vi "cSM.vi"(8 "Error in":errorcluster) -> (0 "Error out":errorcluster)   [LabVIEW 2021, in "EDT VIE.lvlib"]
uses:
  EDT VIE.lvlib
panel:
  out "Current State":string
  out "Previous State":string
  in  "Tab Control":enum32{"Main", "Misc"}(tab)
  out "itr":i32
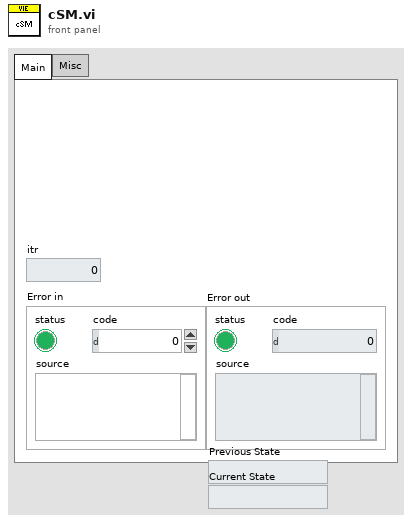
[diagram p1: front panel]
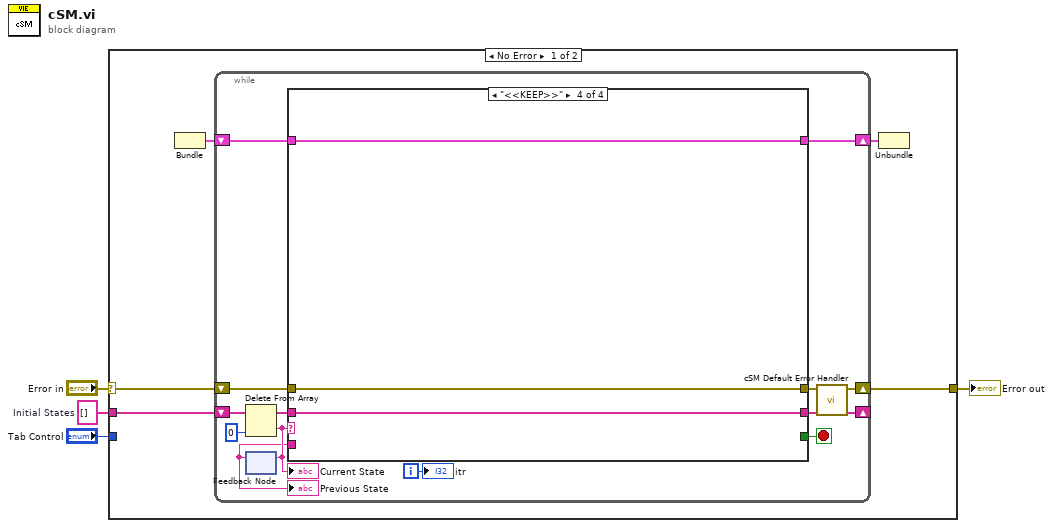
[diagram p0: block diagram]
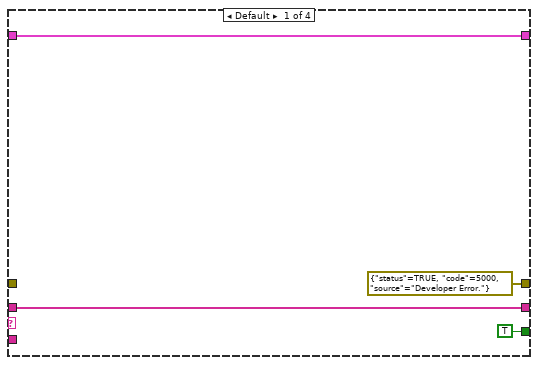
[diagram p2: hidden frame]
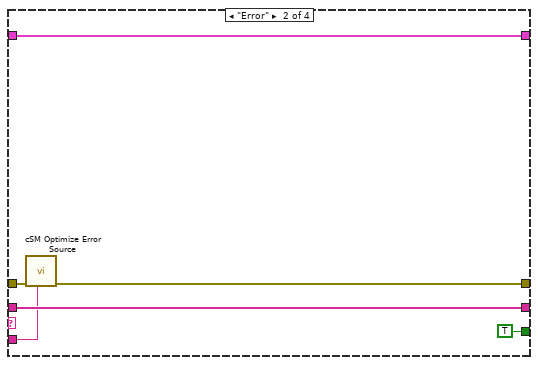
[diagram p3: hidden frame]
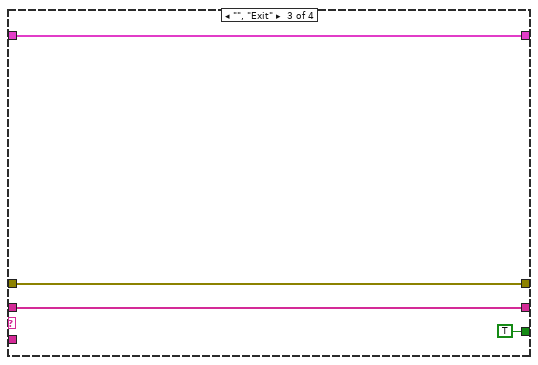
[diagram p4: hidden frame]
diagram:
  w4 = string[] []  # Initial States
  n1 = case shown="No Error" "Error in" {
    selector: "Error in" -> [w7 w41]
    tunnel: w4 -> [w9 _]
    tunnel: [w8 w41] -> w2
    tunnel: "Tab Control" -> [_ _]
    frame No Error {
      n2 = Bundle() -> (w6:cluster{void, void})  [unwired: 3 in]
      n3 = while {
        shift-right: [w10] -> _
        shift-left: w9 -> [w23]
        shift-right: [w12] -> w8
        shift-left: w7 -> [w20]
        shift-right: [w14] -> w5
        shift-left: w6 -> [w15]
        i -> [w21]
        stop <- w19 stop-if-true
        n4 = Delete From Array(array=w23, index=0) -> (deleted portion=w17:string, array with subset deleted=w22:string[])  [unwired: 1 in]
        "Current State" <- w17
        n5 = feedback #1() -> (w16:string)  [unwired: 1 in]
        "Previous State" <- w16
        n6 = feedback-in #1(w17) -> ()
        n7 = case shown="\"<<KEEP>>\"" w17 {
          tunnel: [w25 w33 w37 w40] -> w11
          tunnel: w22 -> [w25 w33 w37 w40]
          tunnel: w20 -> [_ w31 w36 w39]
          tunnel: [errorcluster {"status"=TRUE, "code"=5000, "source"="Developer Error."} ("error in") w30 w36 w39] -> w13
          tunnel: [TRUE TRUE TRUE _] -> w19
          tunnel: w16 -> [_ w29 _ _]
          tunnel: w15 -> [w24 w28 w34 w38]
          tunnel: [w24 w28 w34 w38] -> w14
          frame Default {
          }
          frame "Error" {
            n8 = call "cSM Optimize Error Source.vi"("Previous State"=w29, "Error in"=w31) -> ("Error out"=w30:errorcluster)  [unwired: 9 in]
          }
          frame "", "Exit" {
          }
          frame "<<KEEP>>" {
          }
        }
        n9 = call "cSM Default Error Handler.vi"("States in"=w11, "error in (no error)"=w13) -> ("States out"=w10:string[], "error out"=w12:errorcluster)  [unwired: 8 in]
        "itr" <- w21
      }
      n10 = Unbundle(w5) -> ()  [unwired: 2 out]
    }
    frame Error {
    }
  }
  "Error out" <- w2
